vi "jMsg_TCPConnection_Status (create).vi"(8 "error in (no error)":errorcluster, 11 "Connected?":bool) -> (0 "error out":errorcluster, 3 "jMsg_TCPConnection_Status":refnum<class "jMsg_TCPConnection_Status.lvclass">)   [LabVIEW 2019, in "jMsg_TCPConnection_Status.lvclass"]
doc: "This VI is used to create the jMsg\n\n\nJSMA Message Wizard 0.2.0.5\nRob Humfeld - Jet Engineering\nCopyright (c) 2020, Jet Engineering"
uses:
  jMsg_TCPConnection_Status.lvclass
  C:/Program Files/National Instruments/LabVIEW 2019/user.lib/Jet Engineering/JSMA/Libraries/jMsg Class/jMsg.lvclass
  <userlib>/Jet Engineering/JSMA/Libraries/jMsg Class/jMsg.lvclass/jMsg.ctl
  jMsg_TCPConnection_Status.lvclass/jMsg_TCPConnection_Status.ctl
  <userlib>/Jet Engineering/JSMA/Libraries/Shared/JSMA_GetClassName.vi
  <vilib>/Utility/LVClass/Get LV Class Path.vi
  <userlib>/Jet Engineering/JSMA/Libraries/jMsg Class/jMsg.lvclass
panel:
  in  "jMsg_TCPConnection_Status":refnum<class "jMsg_TCPConnection_Status.lvclass">
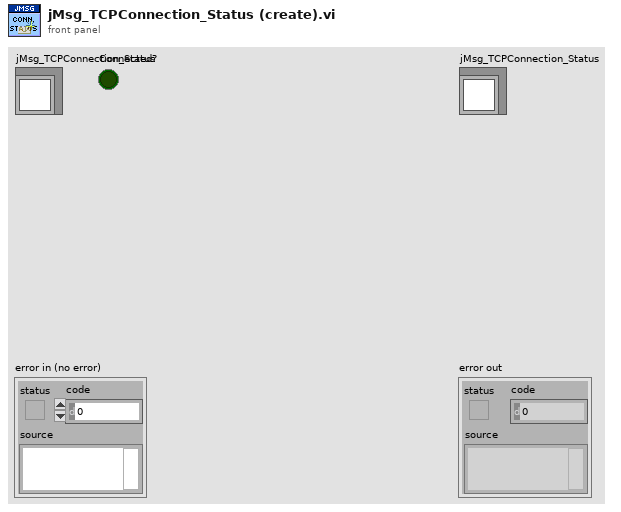
[diagram p1: front panel]
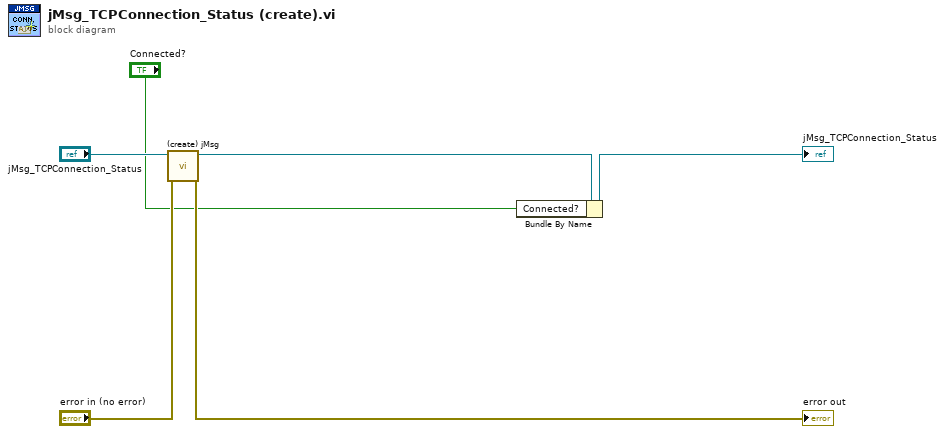
[diagram p0: block diagram]
diagram:
  n1 = call <userlib>:"(create) jMsg.vi"("error in (no error)"="error in (no error)", "jMsg in"="jMsg_TCPConnection_Status") -> ("error out"=→"error out":errorcluster, "jMsg out"=w2:refnum<class "jMsg_TCPConnection_Status.lvclass">)  [unwired: 8 in]
  n2 = Bundle By Name(cluster=w2, "Connected?"="Connected?") -> (→"jMsg_TCPConnection_Status":refnum<class "jMsg_TCPConnection_Status.lvclass">)
